vi "VocmCF_1120.vi"() -> ()   [LabVIEW 2018]
panel:
  in  "Vocm CF(V)":dbl
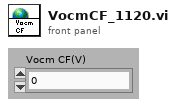
[diagram p1: front panel]
diagram:
